vi "CoPilot Analyze.vi"(0 "JoystickDevRef":T1, 11 "Climbing Manual Enabled":bool) -> (2 "Go Manual":bool, 3 "Flipper Min":bool, 4 "auto shooting management":bool, 6 "Elevation":dbl, 8 "Shoot Motors":dbl, 10 "Flipper Max":bool, 13 "conveyer belt down":bool, 14 "conveyer belt up":bool, 15 "La Fire at will?":bool)   [LabVIEW 2012]
uses:
  <vilib>/Rock Robotics/WPI/Joystick/WPI_JoystickDevRef.ctl
  <vilib>/Rock Robotics/WPI/Joystick/WPI_JoystickDeviceEnum.ctl
  BotStatus.vi
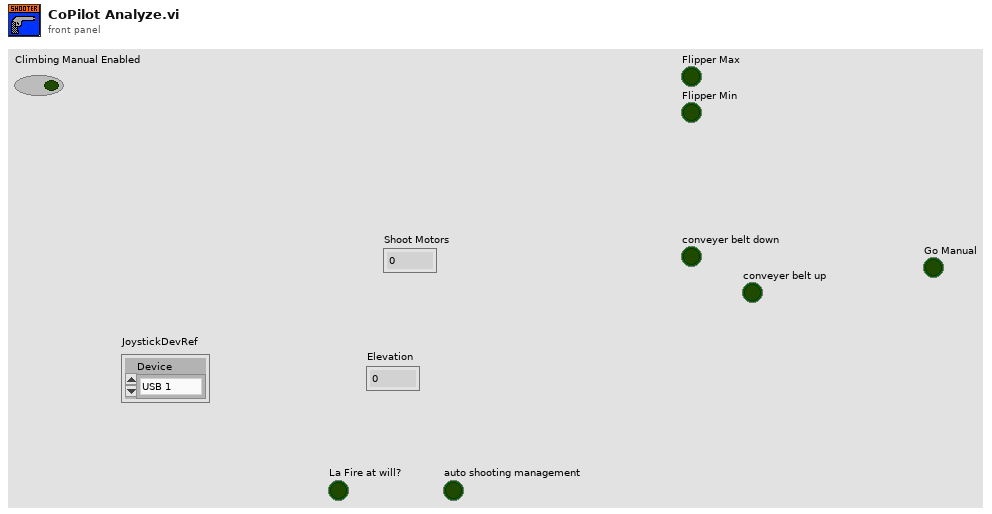
[diagram p1: front panel]
types:
  T1 = typedef "WPI_JoystickDevRef.ctl" = cluster{"Device":T2}
  T2 = typedef "WPI_JoystickDeviceEnum.ctl" = enum16{"USB 1", "USB 2", "USB 3", "USB 4", "Kinect 1", "Kinect 2"}
  T3 = typedef "WPI_JoystickButtonState.ctl" = cluster{"Button 1":bool, "Button 2":bool, "Button 3":bool, "Button 4":bool, "Button 5":bool, "Button 6":bool, "Button 7":bool, "Button 8":bool, "Button 9":bool, "Button 10":bool, "Button 11":bool, "Button 12":bool}
  T4 = cluster{"axis 1 (x)":dbl, "axis 2 (y)":dbl, "axis 3 (throttle)":dbl, "axis 4":dbl, "axis 5":dbl, "axis 6":dbl}
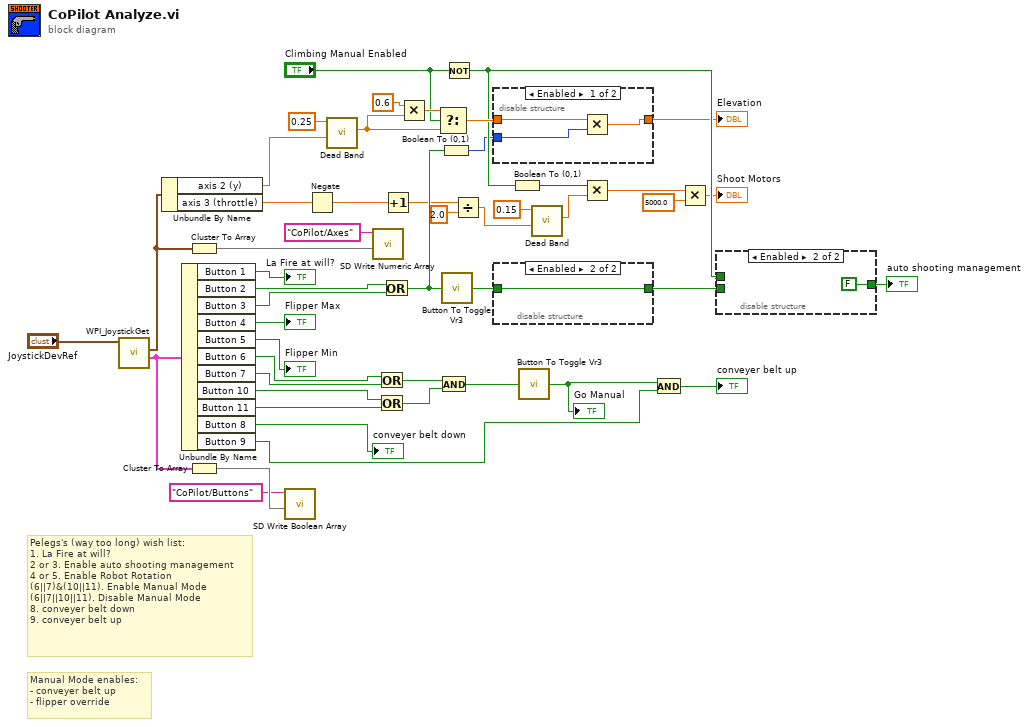
[diagram p0: block diagram]
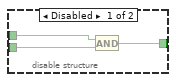
[diagram p3: hidden frame]
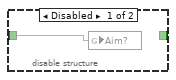
[diagram p4: hidden frame]
diagram:
  # "Manual Mode enables:\n- conveyer belt up\n- flipper override"
  # "Pelegs's (way too long) wish list:\n1. La Fire at will?\n2 or 3. Enable auto shooting management\n4 or 5. Enable Robot Rotation\n(6||7)&(10||11). Enable Manual Mode\n(6||7||10||11). Disable Manual Mode\n8. conveyer belt down\n9. conveyer belt up"
  n1 = call <vilib>:"WPI_JoystickGet.vi"("JoystickDevRef"="JoystickDevRef") -> ("Buttons"=w22:T3, "Axes"=w43:T4)  [unwired: 4 in, 1 out]
  n2 = Unbundle By Name(w43) -> ("axis 2 (y)"=w41:dbl, "axis 3 (throttle)"=w38:dbl)
  n3 = Unbundle By Name(w22) -> ("Button 1"=→"La Fire at will?":bool, "Button 2"=w35:bool, "Button 3"=w34:bool, "Button 4"=→"Flipper Max":bool, "Button 5"=→"Flipper Min":bool, "Button 6"=w33:bool, "Button 7"=w32:bool, "Button 10"=w31:bool, "Button 11"=w30:bool, "Button 8"=→"conveyer belt down":bool, "Button 9"=w24:bool)
  n4 = Cluster To Array(cluster=w43) -> (array=w45:dbl[])
  n5 = Cluster To Array(cluster=w22) -> (array=w47:bool[])
  n6 = call <vilib>:"SD Write Boolean Array.vi"("Boolean Array"=w47, "Name"="CoPilot/Buttons") -> ()  [unwired: 8 in, 2 out]
  n7 = Negate(x=w38) -> (-x=w1:dbl)
  n8 = call "Dead Band.vi"("Axis In"=w41, "Dead Band"=0.25) -> ("Axis Out"=w19:dbl)  [unwired: 9 in]
  n9 = call <vilib>:"SD Write Numeric Array.vi"("Numeric Array"=w45, "Name"="CoPilot/Axes") -> ()  [unwired: 8 in, 2 out]
  n10 = Or(x=w33, y=w32) -> (x .or. y?=w29:bool)
  n11 = Or(x=w31, y=w30) -> (x .or. y?=w28:bool)
  n12 = Or(x=w35, y=w34) -> (x .or. y?=w10:bool)
  n13 = Increment(x=w1) -> (x+1=w3:dbl)
  n14 = Multiply(x=0.6, y=w19) -> (x*y=w20:dbl)
  n15 = Select(t=w20, s="Climbing Manual Enabled", f=w19) -> (s? t:f=w18:dbl)
  n16 = And(x=w29, y=w28) -> (x .and. y?=w8:bool)
  n17 = Boolean To (0,1)(Boolean=w10) -> (0, 1=w9:i16)
  n18 = call "Button To Toggle Vr3.vi"("InValue"=w10) -> ("Result"=w25:bool)
  n19 = Not(x="Climbing Manual Enabled") -> (.not. x?=w14:bool)
  n20 = Divide(x=w3, y=2.0) -> (x/y=w37:dbl)
  n21 = disable-structure shown="Enabled" {
    disable-tunnel: w18 -> [w51 w52]
    disable-tunnel: [w50 w52] -> w11
    disable-tunnel: w9 -> [w49 _]
    frame Enabled {
      n22 = Multiply(x=w51, y=w49) -> (x*y=w50:dbl)
    }
    frame Disabled {
    }
  }
  "Elevation" <- w11
  n23 = disable-structure shown="Enabled" {
    disable-tunnel: w25 -> [w53 w54]
    disable-tunnel: [_ w54] -> w36
    frame Disabled {
      n24 = global write "BotStatus.vi" "Aim?"(w53) -> ()
    }
    frame Enabled {
    }
  }
  n25 = Boolean To (0,1)(Boolean=w14) -> (0, 1=w16:i16)
  n26 = call "Button To Toggle Vr3.vi"("InValue"=w8) -> ("Result"=w7:bool)
  "Go Manual" <- w7
  n27 = call "Dead Band.vi"("Axis In"=w37, "Dead Band"=0.15) -> ("Axis Out"=w26:dbl)  [unwired: 9 in]
  n28 = Multiply(x=w16, y=w26) -> (x*y=w6:dbl)
  n29 = And(x=w7, y=w24) -> (x .and. y?=→"conveyer belt up":bool)
  n30 = Multiply(x=w6, y=5000.0 ("Dead Band")) -> (x*y=→"Shoot Motors":dbl)
  n31 = disable-structure shown="Enabled" {
    disable-tunnel: w36 -> [w57 _]
    disable-tunnel: [w56 FALSE ("auto shooting management")] -> w15
    disable-tunnel: w14 -> [w55 _]
    frame Disabled {
      n32 = And(x=w55, y=w57) -> (x .and. y?=w56:bool)
    }
    frame Enabled {
    }
  }
  "auto shooting management" <- w15
